vi "PH_Sixpack.Motor Type Parameters.vi"(2 "Motor Type":T12) -> (14 "I max [%]":dbl, 16 "Set Stopswitch Limits?":bool, 18 "Stopswitch Limits":T6={"MinLeft(0)"=150, "MaxRight(1023)"=900}, 20 "Set VmaxAmax":bool, 21 "VmaxAmax":T2={"VMax(511)"=511, "AMax(128)"=128}, 22 "Set Axis Parameter":bool, 23 "Axis Parameter":T7={"Poslimit (6400)"=6400, "P5 Bits"={"MT_PI"=FALSE, "MT_ROTARY"=FALSE, "MT_AUTONULLCMD"=FALSE, "MT_TESTNULL"=FALSE, "MT_NULLLEFT"=FALSE, "MT_NULLCENTRE"=TRUE, "MT_STOPNULL"=FALSE, "MT_FILTERSWITCH"=TRUE}, "P6 Bits"={"MT_OPTIMIZEWAY"=FALSE, "MT_FASTREF"=TRUE, "MT_MECHREF"=FALSE, "MT_DELAYTESTNULL"=TRUE, "MT_STOPSOFT"=FALSE, "MT_STOPNOREF"=FALSE, "MT_NULLPOSITIVE"=FALSE, "MUT_STOPFULSTEPS"=FALSE}} {"Poslimit (6400)" step=1}, 24 "Set Ref Search Parameters":bool, 25 "Ref Search Parameters":T5={"VRefMax(100)"=100, "DebouncingTime (22ms)"=34} {"DebouncingTime (22ms)" format="%.0x"}, 27 "6P Axis Config":T1={"VmaxAmax"={"VMax(511)"=511, "AMax(128)"=128}, "I max (50%)"=50.0, "VStartVminDivi"={"VStart(5)"=5, "Vmin(4)"=4, "Div i (2)"=enum."2"}, "Ref Search Parameter"={"VRefMax(100)"=100, "DebouncingTime (22ms)"=34}, "Stopswitch Limits"={"MinLeft(0)"=0, "MaxRight(1023)"=1023}, "Axis Parameter"={"Poslimit (6400)"=6400, "P5 Bits"={"MT_PI"=FALSE, "MT_ROTARY"=FALSE, "MT_AUTONULLCMD"=FALSE, "MT_TESTNULL"=FALSE, "MT_NULLLEFT"=FALSE, "MT_NULLCENTRE"=TRUE, "MT_STOPNULL"=FALSE, "MT_FILTERSWITCH"=TRUE}, "P6 Bits"={"MT_OPTIMIZEWAY"=FALSE, "MT_FASTREF"=TRUE, "MT_MECHREF"=FALSE, "MT_DELAYTESTNULL"=TRUE, "MT_STOPSOFT"=FALSE, "MT_STOPNOREF"=FALSE, "MT_NULLPOSITIVE"=FALSE, "MUT_STOPFULSTEPS"=FALSE}}, "I Control"={"PowerDownDelay (500)"=500, "PowerDown (0%)"=enum."0%", "Standing (50%)"=enum."50%", "Running (75%)"=enum."75%", "Accelerating (100%)"=enum."100%"}} {"Axis Parameter"."Poslimit (6400)" step=1; "Ref Search Parameter"."DebouncingTime (22ms)" format="%.0x"; "I max (50%)" min=0.0 max=100.0})   [LabVIEW 2014, in "PH_Sixpack.lvlib"]
doc: "This VI contains the Motor parameters. The neutral parameter (when the paramter is not set at all) is typically a \"-1\"."
uses:
  PH_Sixpack.lvlib
  instr.lib/SixPack/PackDLL/Ref Search Parameter.ctl
  instr.lib/SixPack/PackDLL/Motor Parameter.ctl
  instr.lib/SixPack/PackDLL/MotorParameter_P5.ctl
  instr.lib/SixPack/PackDLL/MotorParameter_P6.ctl
  instr.lib/SixPack/PackDLL/VmaxAmax.ctl
  instr.lib/SixPack/PackDLL/Stopswitch Limits.ctl
  PH_Stepmotor_BaseClass/PH_Stepmotor_BaseClass.Motor Type.ctl
  PH_Sixpack.Axis Configuration.ctl
  instr.lib/SixPack/PackDLL/PeakCurrent.ctl
  instr.lib/SixPack/PackDLL/VStartVmin.ctl
  instr.lib/SixPack/PackDLL/Current Control.ctl
  instr.lib/SixPack/PackDLL/Current.ctl
  instr.lib/SixPack/Sixpack - Driver.lvlib
  PH_Stepmotor_BaseClass/PH_Stepmotor_BaseClass.lvlib
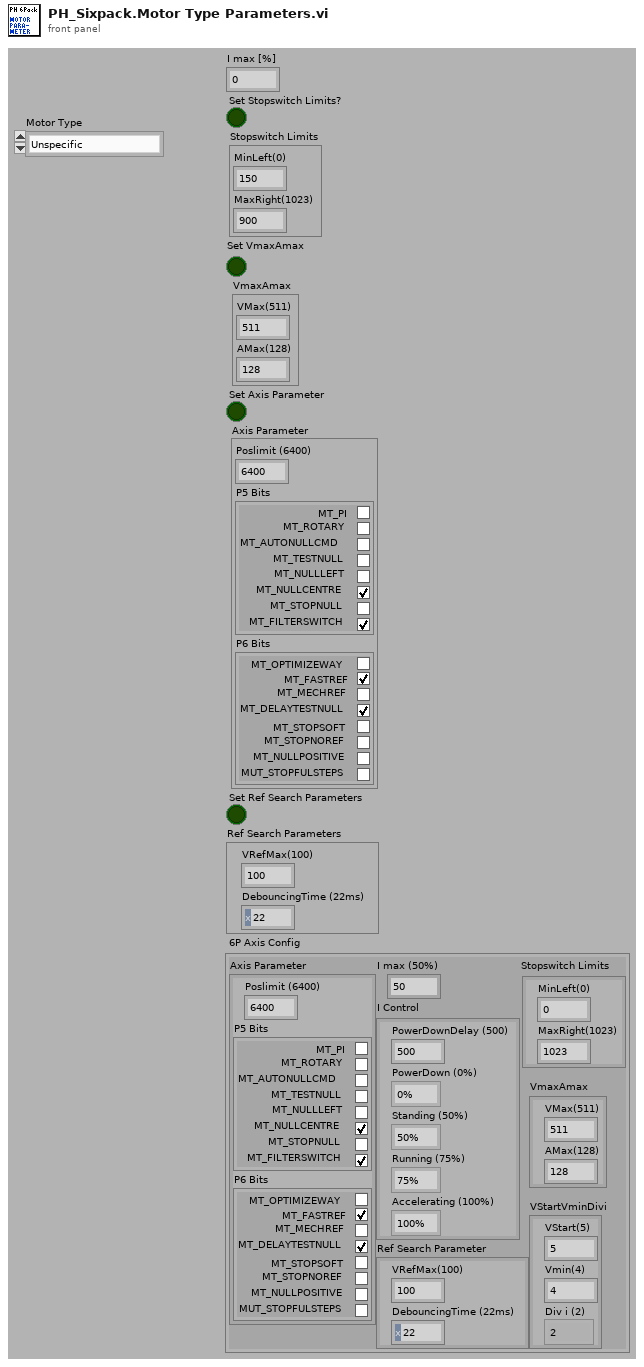
[diagram p1: front panel]
types:
  T1 = typedef "PH_Sixpack.lvlib/PH_Sixpack.Axis Configuration.ctl" = cluster{"VmaxAmax":T2, "I max (50%)":T3, "VStartVminDivi":T4, "Ref Search Parameter":T5, "Stopswitch Limits":T6, "Axis Parameter":T7, "I Control":T10}
  T2 = typedef "Sixpack - Driver.lvlib/VmaxAmax.ctl" = cluster{"VMax(511)":u16, "AMax(128)":u16}
  T3 = typedef "Sixpack - Driver.lvlib/PeakCurrent.ctl" = dbl
  T4 = typedef "Sixpack - Driver.lvlib/VStartVmin.ctl" = cluster{"VStart(5)":u16, "Vmin(4)":u16, "Div i (2)":enum8{"0", "1", "2", "3"}}
  T5 = typedef "Sixpack - Driver.lvlib/Ref Search Parameter.ctl" = cluster{"VRefMax(100)":u16, "DebouncingTime (22ms)":u8}
  T6 = typedef "Sixpack - Driver.lvlib/Stopswitch Limits.ctl" = cluster{"MinLeft(0)":u16, "MaxRight(1023)":u16}
  T7 = typedef "Sixpack - Driver.lvlib/Motor Parameter.ctl" = cluster{"Poslimit (6400)":u32, "P5 Bits":T8, "P6 Bits":T9}
  T8 = typedef "Sixpack - Driver.lvlib/MotorParameter_P5.ctl" = cluster{"MT_PI":bool, "MT_ROTARY":bool, "MT_AUTONULLCMD":bool, "MT_TESTNULL":bool, "MT_NULLLEFT":bool, "MT_NULLCENTRE":bool, "MT_STOPNULL":bool, "MT_FILTERSWITCH":bool}
  T9 = typedef "Sixpack - Driver.lvlib/MotorParameter_P6.ctl" = cluster{"MT_OPTIMIZEWAY":bool, "MT_FASTREF":bool, "MT_MECHREF":bool, "MT_DELAYTESTNULL":bool, "MT_STOPSOFT":bool, "MT_STOPNOREF":bool, "MT_NULLPOSITIVE":bool, "MUT_STOPFULSTEPS":bool}
  T10 = typedef "Sixpack - Driver.lvlib/Current Control.ctl" = cluster{"PowerDownDelay (500)":u16, "PowerDown (0%)":T11, "Standing (50%)":T11, "Running (75%)":T11, "Accelerating (100%)":T11}
  T11 = typedef "Sixpack - Driver.lvlib/Current.ctl" = enum8{"100%", "75%", "50%", "38%", "25%", "19%", "13%", "9%", "0%"}
  T12 = typedef "PH_Stepmotor_BaseClass.lvlib/PH_Stepmotor_BaseClass.Motor Type.ctl" = enum16{"Unspecific", "OWIS 49.120.2633", "OWIS 49.060.1033", "OWIS 43.040.2558", "Diamond Motion 2200 series", "OWIS 49.120.266B.MV6", "Calorimeter", "Linear Stage 1", "MICOS VT-80", "MICOS VT-80 S", "Standa Rotstage nt0.95A", "PUF RA 320.200", "PUF RA 800.200", "PUF RA 800.400", "PUF RA 400.50", "1324.nn.800.50", "1324.n9c.800.50", "1324.nn.320.200", "1324.nn.400.200", "1324.nn.800.200", "1324.nn.400.50", "1324.8c9c.800.50", "1324.8c9c.400.200"}
  T13 = cluster{"Boolean array[0]":bool, "Boolean array[1]":bool, "Boolean array[2]":bool, "Boolean array[3]":bool, "Boolean array[4]":bool, "Boolean array[5]":bool, "Boolean array[6]":bool, "Boolean array[7]":bool}
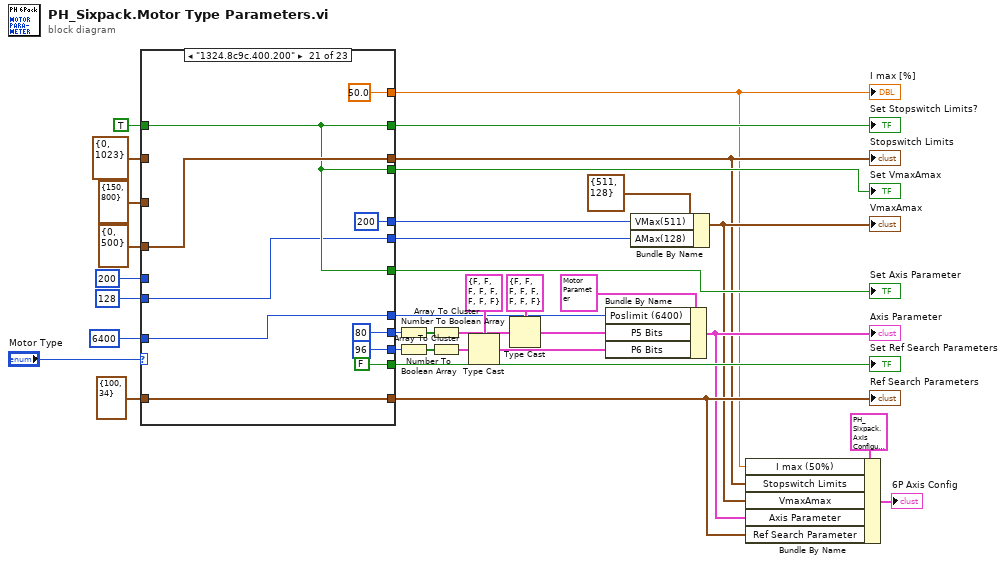
[diagram p0: block diagram]
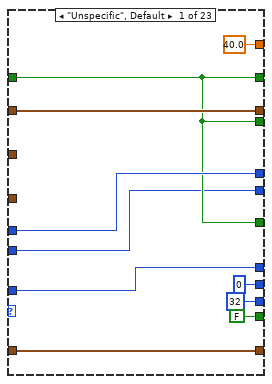
[diagram p2: hidden frame]
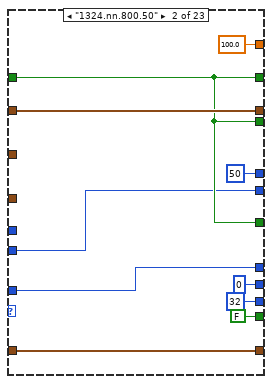
[diagram p3: hidden frame]
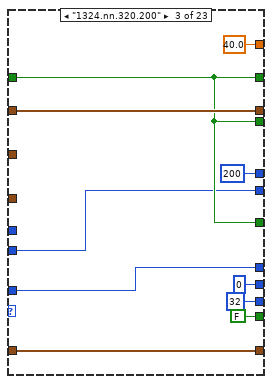
[diagram p4: hidden frame]
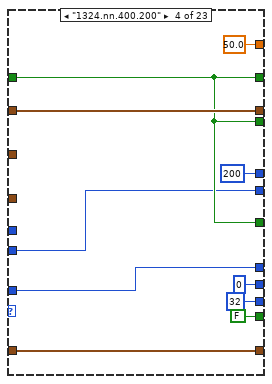
[diagram p5: hidden frame]
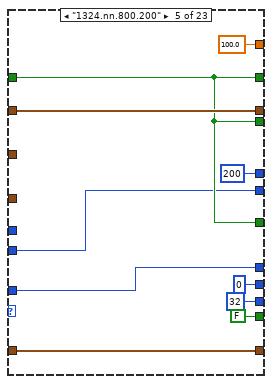
[diagram p6: hidden frame]
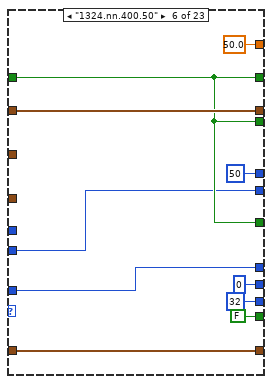
[diagram p7: hidden frame]
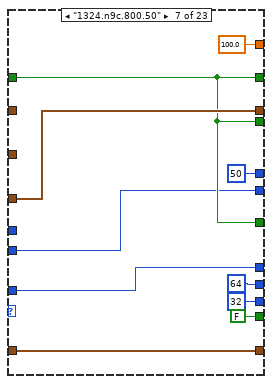
[diagram p8: hidden frame]
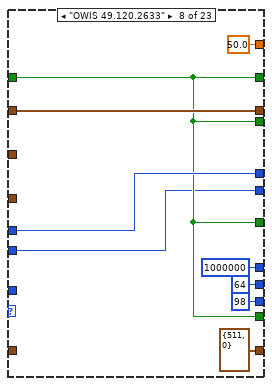
[diagram p9: hidden frame]
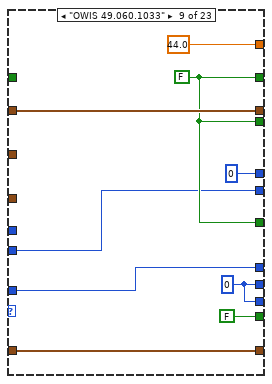
[diagram p10: hidden frame]
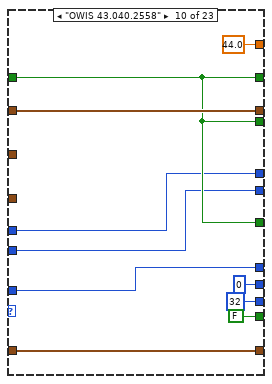
[diagram p11: hidden frame]
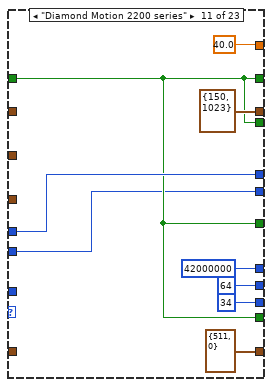
[diagram p12: hidden frame]
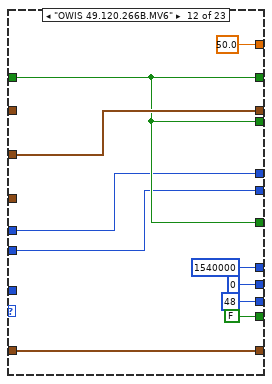
[diagram p13: hidden frame]
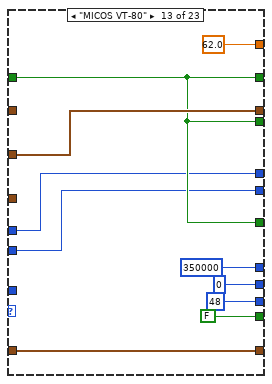
[diagram p14: hidden frame]
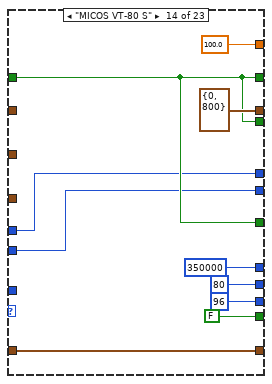
[diagram p15: hidden frame]
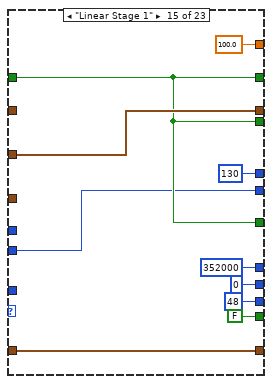
[diagram p16: hidden frame]
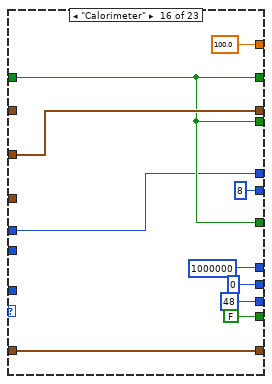
[diagram p17: hidden frame]
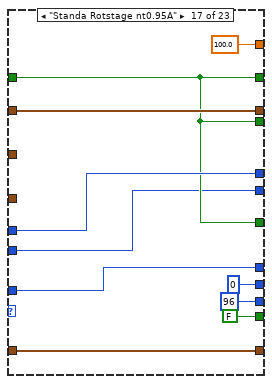
[diagram p18: hidden frame]
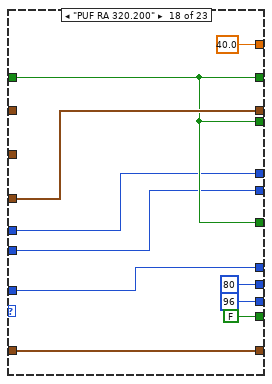
[diagram p19: hidden frame]
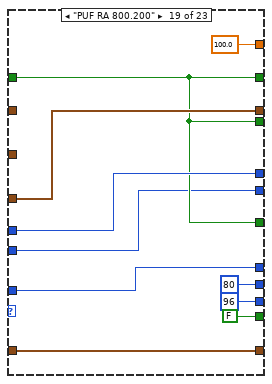
[diagram p20: hidden frame]
diagram:
  n1 = case shown="\"1324.8c9c.400.200\"" "Motor Type" {
    tunnel: [w40 u16 50 ("velocity") u16 200 ("velocity") u16 200 ("velocity") u16 200 ("velocity") u16 50 ("velocity") u16 50 ("velocity") w109 u16 0 ("velocity") w127 w137 w146 w156 w166 u16 130 ("velocity") w186 w197 w206 w217 u16 50 ("velocity") u16 200 ("velocity") u16 400 ("velocity") u16 50 ("velocity")] -> w13
    tunnel: [w41 w50 w60 w70 w80 w90 w100 u32 1000000 ("Poslimit (6400)") w119 w129 u32 42000000 ("Poslimit (6400)") u32 1540000 ("Poslimit (6400)") u32 350000 ("Poslimit (6400)") u32 350000 ("Poslimit (6400)") u32 352000 ("Poslimit (6400)") u32 1000000 ("Poslimit (6400)") w198 w208 w218 w228 w238 w247 w257] -> w17
    tunnel: [u32 32 ("number") u32 32 ("number") u32 32 ("number") u32 32 ("number") u32 32 ("number") u32 32 ("number") u32 32 ("number") u32 98 ("number") w121 u32 32 ("number") u32 34 ("number") u32 48 ("number") u32 48 ("number") u32 96 ("number") u32 48 ("number") u32 48 ("number") u32 96 ("number") u32 96 ("number") u32 96 ("number") u32 96 ("number") u32 96 ("number") u32 96 ("number") u32 96 ("number")] -> w29
    tunnel: [u32 0 ("number") u32 0 ("number") u32 0 ("number") u32 0 ("number") u32 0 ("number") u32 0 ("number") u32 64 ("number") u32 64 ("number") w121 u32 0 ("number") u32 64 ("number") u32 0 ("number") u32 0 ("number") u32 80 ("number") u32 0 ("number") u32 0 ("number") u32 0 ("number") u32 80 ("number") u32 80 ("number") u32 80 ("number") u32 80 ("number") u32 80 ("number") u32 80 ("number")] -> w30
    tunnel: [w38 w47 w57 w67 w77 w87 w97 T5 {"VRefMax(100)"=511, "DebouncingTime (22ms)"=0} ("Ref Search Parameters") w116 w125 T5 {"VRefMax(100)"=511, "DebouncingTime (22ms)"=0} ("Ref Search Parameters") w144 w154 w165 w174 w185 w195 w204 w215 w226 w236 w245 w254] -> w5
    tunnel: [FALSE ("Bit 0: PI Mode (FALSE)") FALSE ("Bit 0: PI Mode (FALSE)") FALSE ("Bit 0: PI Mode (FALSE)") FALSE ("Bit 0: PI Mode (FALSE)") FALSE ("Bit 0: PI Mode (FALSE)") FALSE ("Bit 0: PI Mode (FALSE)") FALSE ("Bit 0: PI Mode (FALSE)") w108 FALSE ("Bit 0: PI Mode (FALSE)") FALSE ("Bit 0: PI Mode (FALSE)") w135 FALSE ("Bit 0: PI Mode (FALSE)") FALSE ("Bit 0: PI Mode (FALSE)") FALSE ("Bit 0: PI Mode (FALSE)") FALSE ("Bit 0: PI Mode (FALSE)") FALSE ("Bit 0: PI Mode (FALSE)") FALSE ("Bit 0: PI Mode (FALSE)") FALSE ("Bit 0: PI Mode (FALSE)") FALSE ("Bit 0: PI Mode (FALSE)") FALSE ("Bit 0: PI Mode (FALSE)") FALSE ("Bit 0: PI Mode (FALSE)") FALSE ("Bit 0: PI Mode (FALSE)") FALSE ("Bit 0: PI Mode (FALSE)")] -> w31
    tunnel: [40.0 ("I max (200)") 100.0 ("I max (200)") 40.0 ("I max (200)") 50.0 ("I max (200)") 100.0 ("I max (200)") 50.0 ("I max (200)") 100.0 ("I max (200)") 50.0 ("I max (200)") 44.0 ("I max (200)") 44.0 ("I max (200)") 40.0 ("I max (200)") 50.0 ("I max (200)") 62.0 ("I max (200)") 100.0 ("I max (200)") 100.0 ("I max (200)") 100.0 ("I max (200)") 100.0 ("I max (200)") 40.0 ("I max (200)") 100.0 ("I max (200)") 100.0 ("I max (200)") 50.0 ("I max (200)") 100.0 ("I max (200)") 50.0 ("I max (200)")] -> w1
    tunnel: [w39 w49 w59 w69 w79 w89 w99 w108 w118 w128 w135 w147 w157 w167 w176 w187 w196 w207 w216 w227 w237 w246 w256] -> w24
    tunnel: TRUE -> [w39 w49 w59 w69 w79 w89 w99 w108 _ w128 w135 w147 w157 w167 w176 w187 w196 w207 w216 w227 w237 w246 w256]
    tunnel: [w43 w51 w61 w71 w81 w91 w101 w110 w120 w130 T6 {"MinLeft(0)"=150, "MaxRight(1023)"=1023} ("Stopswitch Limits") w148 w158 T6 {"MinLeft(0)"=0, "MaxRight(1023)"=800} ("Stopswitch Limits") w177 w188 w199 w209 w219 w229 w239 w248 w258] -> w2
    tunnel: T6 {"MinLeft(0)"=0, "MaxRight(1023)"=1023} ("Stopswitch Limits") -> [w43 w51 w61 w71 w81 w91 _ w110 w120 w130 _ _ _ _ _ _ w199 _ _ _ _ _ _]
    tunnel: T6 {"MinLeft(0)"=150, "MaxRight(1023)"=800} ("Stopswitch Limits") -> [_ _ _ _ _ _ _ _ _ _ _ w148 w158 _ w177 w188 _ _ _ _ _ _ _]
    tunnel: T6 {"MinLeft(0)"=0, "MaxRight(1023)"=500} ("Stopswitch Limits") -> [_ _ _ _ _ _ w101 _ _ _ _ _ _ _ _ _ _ w209 w219 w229 w239 w248 w258]
    tunnel: [w39 w49 w59 w69 w79 w89 w99 w108 w118 w128 w135 w147 w157 w167 w176 w187 w196 w207 w216 w227 w237 w246 w256] -> w20
    tunnel: u32 6400 ("Poslimit (6400)") -> [w41 w50 w60 w70 w80 w90 w100 _ w119 w129 _ _ _ _ _ _ w198 w208 w218 w228 w238 w247 w257]
    tunnel: [w39 w49 w59 w69 w79 w89 w99 w108 w118 w128 w135 w147 w157 w167 w176 w187 w196 w207 w216 w227 w237 w246 w256] -> w14
    tunnel: u16 200 ("velocity") -> [w40 _ _ _ _ _ _ w109 _ w127 w137 w146 w156 w166 _ w186 w197 w206 w217 _ _ _ _]
    tunnel: T5 {"VRefMax(100)"=100, "DebouncingTime (22ms)"=34} ("Ref Search Parameters") -> [w38 w47 w57 w67 w77 w87 w97 _ w116 w125 _ w144 w154 w165 w174 w185 w195 w204 w215 w226 w236 w245 w254]
    tunnel: [w36 w46 w56 w66 w76 w86 w96 w106 w115 w124 w134 w143 w153 w163 w173 u16 8 ("AMax(128)") w193 w203 w213 w224 w234 w243 w253] -> w9
    tunnel: u16 128 ("AMax(128)") -> [w36 w46 w56 w66 w76 w86 w96 w106 w115 w124 w134 w143 w153 w163 w173 _ w193 w203 w213 w224 w234 w243 w253]
    frame "Unspecific", Default {
    }
    frame "1324.nn.800.50" {
    }
    frame "1324.nn.320.200" {
    }
    frame "1324.nn.400.200" {
    }
    frame "1324.nn.800.200" {
    }
    frame "1324.nn.400.50" {
    }
    frame "1324.n9c.800.50" {
    }
    frame "OWIS 49.120.2633" {
    }
    frame "OWIS 49.060.1033" {
      w118 = FALSE
      w121 = u32 0 ("number")
    }
    frame "OWIS 43.040.2558" {
    }
    frame "Diamond Motion 2200 series" {
    }
    frame "OWIS 49.120.266B.MV6" {
    }
    frame "MICOS VT-80" {
    }
    frame "MICOS VT-80 S" {
    }
    frame "Linear Stage 1" {
    }
    frame "Calorimeter" {
    }
    frame "Standa Rotstage nt0.95A" {
    }
    frame "PUF RA 320.200" {
    }
    frame "PUF RA 800.200" {
    }
    frame "1324.8c9c.800.50" {
    }
    frame "1324.8c9c.400.200" {
    }
    frame "PUF RA 800.400" {
    }
    frame "PUF RA 400.50" {
    }
  }
  "I max [%]" <- w1
  "Set Ref Search Parameters" <- w31
  "Ref Search Parameters" <- w5
  "Set Axis Parameter" <- w20
  "Set Stopswitch Limits?" <- w24
  "Stopswitch Limits" <- w2
  "Set VmaxAmax" <- w14
  n2 = Number To Boolean Array(number=w30) -> (Boolean array=w27:bool[])
  n3 = Number To Boolean Array(number=w29) -> (Boolean array=w35:bool[])
  n4 = Array To Cluster(array=w27) -> (cluster=w28:T13)
  n5 = Array To Cluster(array=w35) -> (cluster=w34:T13)
  n6 = Type Cast(type=T9 {"MT_OPTIMIZEWAY"=FALSE, "MT_FASTREF"=FALSE, "MT_MECHREF"=FALSE, "MT_DELAYTESTNULL"=FALSE, "MT_STOPSOFT"=FALSE, "MT_STOPNOREF"=FALSE, "MT_NULLPOSITIVE"=FALSE, "MUT_STOPFULSTEPS"=FALSE} ("P6 Bits"), x=w34) -> (*(type *) &x=w19:T9)
  n7 = Type Cast(type=T8 {"MT_PI"=FALSE, "MT_ROTARY"=FALSE, "MT_AUTONULLCMD"=FALSE, "MT_TESTNULL"=FALSE, "MT_NULLLEFT"=FALSE, "MT_NULLCENTRE"=FALSE, "MT_STOPNULL"=FALSE, "MT_FILTERSWITCH"=FALSE} ("P5 Bits"), x=w28) -> (*(type *) &x=w18:T8)
  n8 = Bundle By Name(cluster=T7 {"Poslimit (6400)"=6400, "P5 Bits"={"MT_PI"=FALSE, "MT_ROTARY"=FALSE, "MT_AUTONULLCMD"=FALSE, "MT_TESTNULL"=FALSE, "MT_NULLLEFT"=FALSE, "MT_NULLCENTRE"=TRUE, "MT_STOPNULL"=FALSE, "MT_FILTERSWITCH"=TRUE}, "P6 Bits"={"MT_OPTIMIZEWAY"=FALSE, "MT_FASTREF"=TRUE, "MT_MECHREF"=FALSE, "MT_DELAYTESTNULL"=TRUE, "MT_STOPSOFT"=FALSE, "MT_STOPNOREF"=FALSE, "MT_NULLPOSITIVE"=FALSE, "MUT_STOPFULSTEPS"=FALSE}} ("Axis Parameter"), "Poslimit (6400)"=w17, "P5 Bits"=w18, "P6 Bits"=w19) -> (w4:T7)
  "Axis Parameter" <- w4
  n9 = Bundle By Name(cluster=T2 {"VMax(511)"=511, "AMax(128)"=128} ("V max A max"), "VMax(511)"=w13, "AMax(128)"=w9) -> (w3:T2)
  "VmaxAmax" <- w3
  n10 = Bundle By Name(cluster=T1 {"VmaxAmax"={"VMax(511)"=511, "AMax(128)"=128}, "I max (50%)"=50.0, "VStartVminDivi"={"VStart(5)"=5, "Vmin(4)"=4, "Div i (2)"=enum."2"}, "Ref Search Parameter"={"VRefMax(100)"=100, "DebouncingTime (22ms)"=34}, "Stopswitch Limits"={"MinLeft(0)"=0, "MaxRight(1023)"=1023}, "Axis Parameter"={"Poslimit (6400)"=6400, "P5 Bits"={"MT_PI"=FALSE, "MT_ROTARY"=FALSE, "MT_AUTONULLCMD"=FALSE, "MT_TESTNULL"=FALSE, "MT_NULLLEFT"=FALSE, "MT_NULLCENTRE"=TRUE, "MT_STOPNULL"=FALSE, "MT_FILTERSWITCH"=TRUE}, "P6 Bits"={"MT_OPTIMIZEWAY"=FALSE, "MT_FASTREF"=TRUE, "MT_MECHREF"=FALSE, "MT_DELAYTESTNULL"=TRUE, "MT_STOPSOFT"=FALSE, "MT_STOPNOREF"=FALSE, "MT_NULLPOSITIVE"=FALSE, "MUT_STOPFULSTEPS"=FALSE}}, "I Control"={"PowerDownDelay (500)"=500, "PowerDown (0%)"=enum."0%", "Standing (50%)"=enum."50%", "Running (75%)"=enum."75%", "Accelerating (100%)"=enum."100%"}} ("6P Axis Config"), "I max (50%)"=w1, "Stopswitch Limits"=w2, "VmaxAmax"=w3, "Axis Parameter"=w4, "Ref Search Parameter"=w5) -> (→"6P Axis Config":T1)
